vi "2.Bounce Window_Data Management.vi"(11 "群組：":T1) -> (3 "資料管理選單":T2)   [LabVIEW 2015]
uses:
  0.Main_Control/Control_Bounce Window_Main_Data Management.ctl
  <vilib>/Utility/miscctls.llb/LVPointTypeDef.ctl
panel:
  in  "離開":bool
  in  "操作履歷":bool
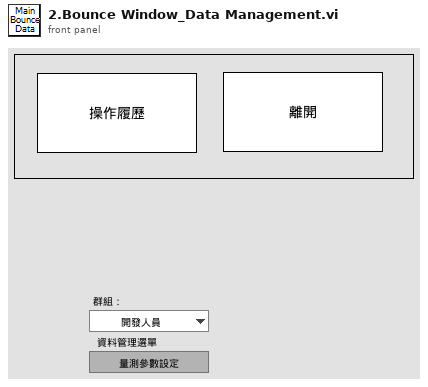
[diagram p1: front panel]
types:
  T1 = typedef "Control_User account_Permissions.ctl" = enum16{"開發人員", "管理者", "工程師", "作業員"}
  T2 = typedef "Control_Bounce Window_Main_Data Management.ctl" = enum16{"量測參數設定", "操作履歷", "數據回顧", "離開", "等待"}
  T3 = typedef "LVPointTypeDef.ctl" = cluster{"Horizontal":i16, "Vertical":i16}
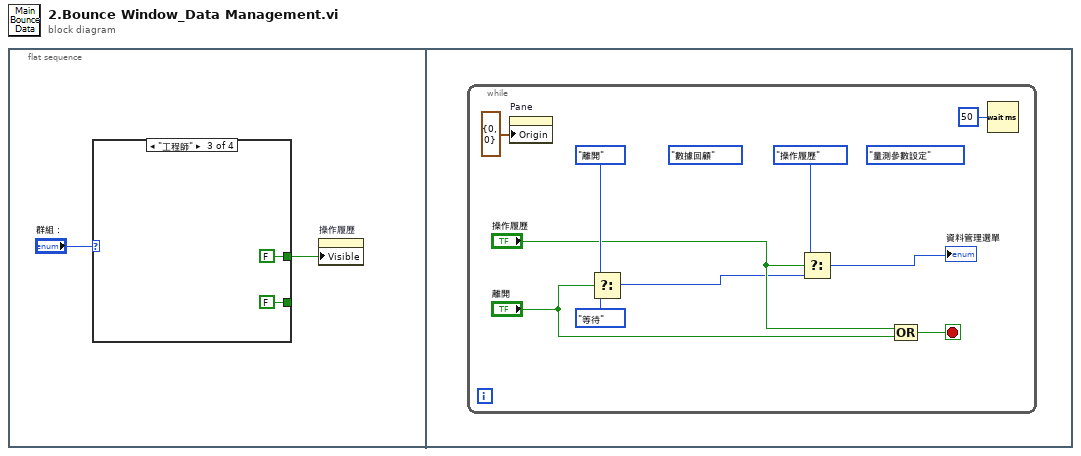
[diagram p0: block diagram]
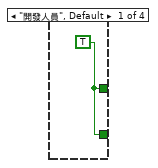
[diagram p2: hidden frame]
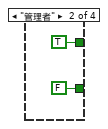
[diagram p3: hidden frame]
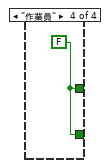
[diagram p4: hidden frame]
diagram:
  n1 = flat-sequence {
    frame #0 {
      n2 = case shown="\"工程師\"" "群組：" {
        tunnel: [w3 FALSE FALSE w8] -> _
        tunnel: [w3 TRUE FALSE w8] -> w1
        frame "開發人員", Default {
          w3 = TRUE
        }
        frame "管理者" {
        }
        frame "工程師" {
        }
        frame "作業員" {
          w8 = FALSE
        }
      }
      n3 = property on="操作履歷" class="Bool"("Visible"=w1) -> ()  [unwired: 2 in, 2 out]
    }
    frame #1 {
      n4 = while {
        stop <- w14 stop-if-true
        (unwired) Control_Bounce_Window_Main_Data_Management."數據回顧" ("資料管理選單")
        (unwired) Control_Bounce_Window_Main_Data_Management."量測參數設定" ("資料管理選單")
        n5 = property on="Pane" class="Pane"("Origin"=T3 {"Horizontal"=0, "Vertical"=0}) -> ()  [unwired: 2 in, 2 out]
        n6 = Select(t=Control_Bounce_Window_Main_Data_Management."離開" ("資料管理選單"), s="離開", f=Control_Bounce_Window_Main_Data_Management."等待" ("資料管理選單")) -> (s? t:f=w10:T2)
        n7 = Select(t=Control_Bounce_Window_Main_Data_Management."操作履歷" ("資料管理選單"), s="操作履歷", f=w10) -> (s? t:f=→"資料管理選單":T2)
        n8 = Compound Arithmetic op=OR("操作履歷", "離開") -> (w14:bool)
        n9 = Wait (ms)(milliseconds to wait=u32 50) -> ()  [unwired: 1 out]
      }
    }
  }
